vi "Read String.vi"(8 "error in (no error)":errorcluster, 11 "NI Analog in":refnum<class "NI Digital to Analog.lvclass">) -> (0 "error out":errorcluster, 1 "Bytes Read":i32, 2 "String Read":string, 3 "NI Analog out":refnum<class "NI Digital to Analog.lvclass">)   [LabVIEW 2024, in "NI Digital to Analog.lvclass"]
doc: "Bus.lvclass:Read String.vi\n\nThis is the template for the Read String VI forthe Bus class.\n\nInstrument Communication Module Version 1.0\nJuly, 2017 Original Code Consulting David Thomson\n www.originalcode.com"
uses:
  NI Digital to Analog.lvclass
  NI Digital to Analog.lvclass/NI Digital to Analog.ctl
  <vilib>/DAQmx/read.llb/DAQmx Read (Analog 1D DBL NChan 1Samp).vi
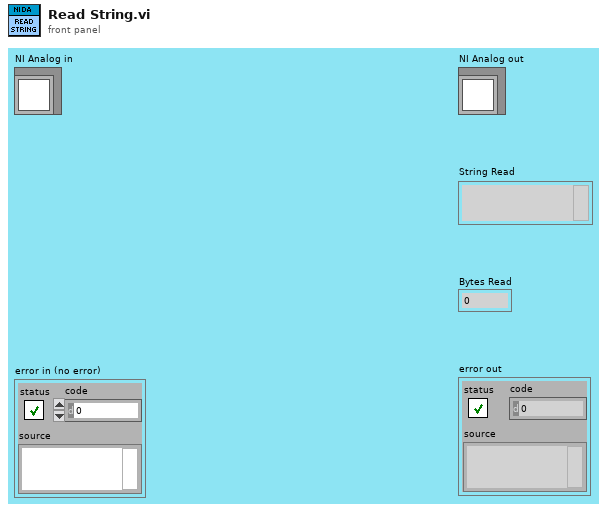
[diagram p1: front panel]
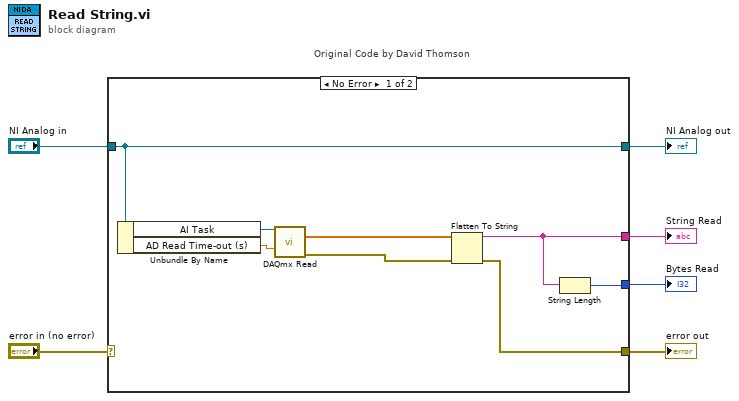
[diagram p0: block diagram]
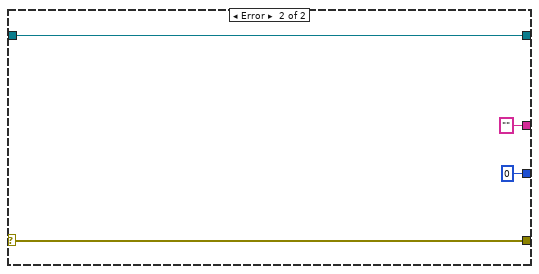
[diagram p2: hidden frame]
diagram:
  n1 = case "Original Code by David Thomson" shown="No Error" "error in (no error)" {
    selector: "error in (no error)" -> [_ w18]
    tunnel: [w9 w18] -> w5
    tunnel: [w13 w17] -> w4
    tunnel: "NI Analog in" -> [w13 w17]
    tunnel: [w8 ""] -> w2
    tunnel: [w7 0] -> w1
    frame No Error {
      n2 = Unbundle By Name(w13) -> ("AI Task"=w14:refnum<k21>, "AD Read Time-out (s)"=w12:dbl)
      n3 = call-poly <vilib>:"DAQmx Read.vi"("task/channels in"=w14, "timeout"=w12) -> ("data"=w11:dbl[], "error out"=w10:errorcluster)  [unwired: 11 in, 1 out]
      n4 = Flatten To String(anything=w11, error in (no error)=w10) -> (data string=w8:string, error out=w9:errorcluster)  [unwired: 2 in, 1 out]
      n5 = String Length(string=w8) -> (length=w7:i32)
    }
    frame Error {
    }
  }
  "error out" <- w5
  "NI Analog out" <- w4
  "Bytes Read" <- w1
  "String Read" <- w2
